vi "Write All Elements Hidden.vi"(8 "error in (no error)":errorcluster, 10 "Analys. params. hidden":T1={"Melt-pool connectivity"=TRUE, "Melt-pool characteristics"=[35, 22, 25]} {"Melt-pool characteristics" items=["Center of Mass X", "Center of Mass Y", "First Pixel X", "First Pixel Y", "Bounding Rect Left", "Bounding Rect Top", "Bounding Rect Right", "Bounding Rect Bottom", "Max Feret Diameter Start X", "Max Feret Diameter Start Y", "Max Feret Diameter End X", "Max Feret Diameter End Y", "Max Horiz. Segment Length Left", "Max Horiz. Segment Length Right", "Max Horiz. Segment Length Row", "-", "Bounding Rect Width", "Bounding Rect Height", "Bounding Rect Diagonal", "Perimeter", "Convex Hull Perimeter", "Holes' Perimeter", "Max Feret Diameter", "Equivalent Ellipse Major Axis", "Equivalent Ellipse Minor Axis", "Equivalent Ellipse Minor Axis (Feret)", "Equivalent Rect Long Side", "Equivalent Rect Short Side", "Equivalent Rect Diagonal", "Equivalent Rect Short Side (Feret)", "Average Horiz. Segment Length", "Average Vert. Segment Length", "Hydraulic Radius", "Waddel Disk Diameter", "-", "Area", "Holes' Area", "Particle & Holes' Area", "Convex Hull Area", "Image Area", "-", "Number of Holes", "Number of Horiz. Segments", "Number of Vert. Segments", "-", "Orientation", "Max Feret Diameter Orientation", "-", "% Area/Image Area", "% Area/(Particle & Holes' Area)", "Ratio of Equivalent Ellipse Axes", "Ratio of Equivalent Rect Sides", "-", "Elongation Factor", "Compactness Factor", "Heywood Circularity Factor", "Type Factor", "-", "Sum X", "Sum Y", "Sum XX", "Sum XY", "Sum YY", "Sum XXX", "Sum XXY", "Sum XYY", "Sum YYY", "-", "Moment of Inertia XX", "Moment of Inertia XY", "Moment of Inertia YY", "Moment of Inertia XXX", "Moment of Inertia XXY", "Moment of Inertia XYY", "Moment of Inertia YYY", "Norm. Moment of Inertia XX", "Norm. Moment of Inertia XY", "Norm. Moment of Inertia YY", "Norm. Moment of Inertia XXX", "Norm. Moment of Inertia XXY", "Norm. Moment of Inertia XYY", "Norm. Moment of Inertia YYY", "Hu Moment 1", "Hu Moment 2", "Hu Moment 3", "Hu Moment 4", "Hu Moment 5", "Hu Moment 6", "Hu Moment 7"]}, 11 "Analysis params in":refnum<class "CV-Analysis.lvclass">) -> (0 "error out":errorcluster, 3 "Analysis params out":refnum<class "CV-Analysis.lvclass">)   [LabVIEW 2013, in "CameraVision.lvlib" / "CV-Analysis.lvclass"]
uses:
  CV-Analysis.lvclass
  Analysis-parameters-advanced.ctl
  CV-Analysis.lvclass/CV-Analysis.ctl
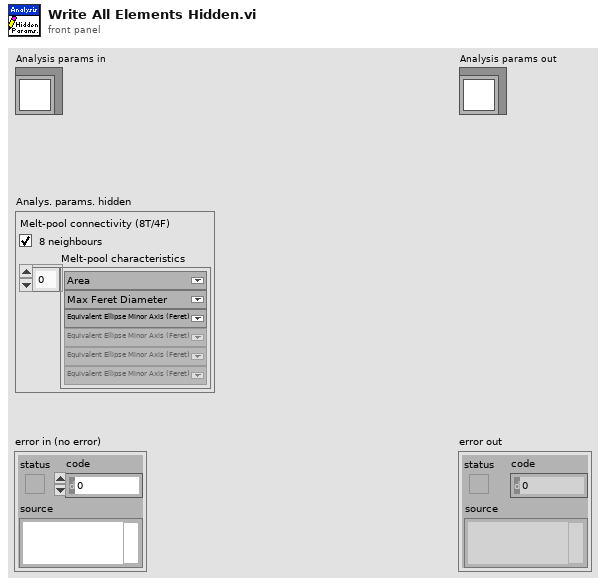
[diagram p1: front panel]
types:
  T1 = typedef "CameraVision.lvlib/CV-Analysis.lvclass/Analysis-parameters-advanced.ctl" = cluster{"Melt-pool connectivity":bool, "Melt-pool characteristics":T2[]}
  T2 = typedef "Particle Parameters" = i32
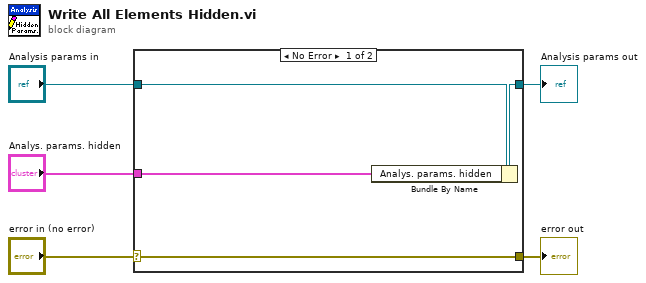
[diagram p0: block diagram]
diagram:
  n1 = case shown="No Error" "error in (no error)" {
    selector: "error in (no error)" -> [w9 w10]
    tunnel: [w9 w10] -> w4
    tunnel: [w7 w11] -> w2
    tunnel: "Analysis params in" -> [w8 w11]
    tunnel: "Analys. params. hidden" -> [w6 _]
    frame No Error {
      n2 = Bundle By Name(cluster=w8, "Analys. params. hidden"=w6) -> (w7:refnum<class "CV-Analysis.lvclass">)
    }
    frame Error {
    }
  }
  "error out" <- w4
  "Analysis params out" <- w2
